vi "Teleop.vi"(10 "Match Info":T1={"Autonomous Elapsed Seconds"=0.0, "TeleOp Elapsed Seconds"=0.0, "Disabled Elapsed Seconds"=0.0, "Visited Autonomous"=FALSE, "Visited TeleOp"=FALSE, "Visited Disabled"=FALSE, "Autonomous Settings"={"Autonomous Style"=enum."Independent", "VI Refnum"=refnum}}, 11 "Call Context":T2) -> ()   [LabVIEW 2020]
doc: "This VI is called for each TeleOp packet received from the DS where the robot is not disabled. It is often used to read from the joysticks and update I/O or to update setpoints for timed control loops. It should complete and return within 20 milliseconds or it may miss DS packets."
uses:
  <vilib>/Rock Robotics/WPI/DriverStation/WPI_DriverStationDerivedRobotMode.ctl
  <vilib>/Rock Robotics/WPI/DriverStation/WPI_DriverStationMatch Info.ctl
  <vilib>/Rock Robotics/WPI/ThirdParty/Phoenix-LabVIEW/Motor Controller/Controls/CTRE_Phoenix_MotorControl_ControlMode.ctl
  <vilib>/Rock Robotics/Network Tables/NT Write Boolean.vi
  <vilib>/Rock Robotics/Network Tables/NT Read Boolean.vi
  <vilib>/Rock Robotics/Network Tables/NT Read Number.vi
  <vilib>/Rock Robotics/WPI/Utilities/WPI_GetSetVariantRefNum.vi
  TitanLib/Lib/Piston Hold.vi
  <vilib>/Rock Robotics/WPI/Solenoid/WPI_SolenoidSetEnum.vi
  TitanLib/Lib/TitanLib.lvlib
panel:
  out "Sample Slider 0":dbl(slide) scale=0.0..5.0
  out "Sample Boolean 1":bool
  out "Sample Boolean 0":bool
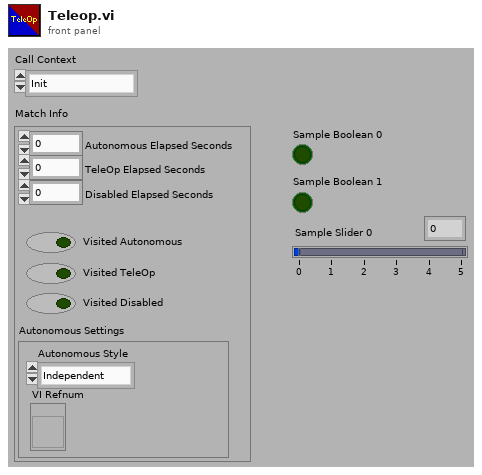
[diagram p1: front panel]
types:
  T1 = typedef "WPI_DriverStationMatch Info.ctl" = cluster{"Autonomous Elapsed Seconds":dbl, "TeleOp Elapsed Seconds":dbl, "Disabled Elapsed Seconds":dbl, "Visited Autonomous":bool, "Visited TeleOp":bool, "Visited Disabled":bool, "Autonomous Settings":cluster{"Autonomous Style":enum16{"Iterative", "Independent"}, "VI Refnum":refnum<vi>}}
  T2 = typedef "WPI_DriverStationDerivedRobotMode.ctl" = enum16{"Init", "Execute", "Stop"}
  T3 = typedef "CTRE_Phoenix_MotorControl_ControlMode.ctl" = u16
  T4 = typedef "WPI_DigitalInputDevRef.ctl" = cluster{"DevStatus":errorcluster, "DIO Channel":T5}
  T5 = typedef "FPGA_DIOChannel.ctl" = enum8{"DIO 0", "DIO 1", "DIO 2", "DIO 3", "DIO 4", "DIO 5", "DIO 6", "DIO 7", "DIO 8", "DIO 9", "DIO MXP 0", "DIO MXP 1", "DIO MXP 2", "DIO MXP 3", "DIO MXP 4", "DIO MXP 5", "DIO MXP 6", "DIO MXP 7", "DIO MXP 8", "DIO MXP 9", "DIO MXP 10", "DIO MXP 11", "DIO MXP 12", "DIO MXP 13", "DIO MXP 14", "DIO MXP 15", "SPI Port CS1", "SPI Port CS2", "SPI Port CS3", "SPI Port MISO", "SPI Port MOSI", "Invalid"}
  T6 = typedef "WPI_JoystickDevRef.ctl" = cluster{"Device":T7}
  T7 = typedef "WPI_JoystickDeviceEnum.ctl" = enum16{"USB 0", "USB 1", "USB 2", "USB 3", "USB 4", "USB 5"}
  T8 = typedef "WPI_MotorControlDeviceRef.ctl" = cluster{"DeviceStatus":errorcluster, "Type":T9, "PWM":cluster{"PWM Channel":T10, "DeadBand":T11}, "CAN":cluster{"Device Number":u8, "SetOutput VI Ref":variant, "GetOutput VI Ref":variant, "Enable VI Ref":variant, "Disable VI Ref":variant, "Data":variant}, "Invert":bool, "DIO PWM":cluster{"PWM \"Enable\" Channel":T10, "DIOChannel":T5, "PWM Rate":dbl}}
  T9 = typedef "WPI_MotorControlType.ctl" = enum16{"PWM", "CAN", "DIO PWM"}
  T10 = typedef "FPGA_DIOPWMChannel.ctl" = enum8{"PWM 0", "PWM 1", "PWM 2", "PWM 3", "PWM 4", "PWM 5", "PWM 6", "PWM 7", "PWM 8", "PWM 9", "PWM MXP 0", "PWM MXP 1", "PWM MXP 2", "PWM MXP 3", "PWM MXP 4", "PWM MXP 5", "PWM MXP 6", "PWM MXP 7", "PWM MXP 8", "PWM MXP 9", "Invalid"}
  T11 = typedef "WPI_PWMDeadband.ctl" = cluster{"Name":string, "maxPositivePwm":i32, "minPositivePwm":i32, "centerPwm":i32, "maxNegativePwm":i32, "minNegativePwm":i32, "angularRange":u16}
  T12 = typedef "WPI_SolenoidValue.ctl" = enum16{"Off", "On", "Forward", "Reverse"}
  T13 = typedef "WPI_SolenoidDevRef.ctl" = cluster{"DevStatus":errorcluster, "Pneumatics Control Module":u8, "Forward Solenoid Channel":T14, "Reverse Solenoid Channel":T14}
  T14 = typedef "WPI_SolenoidChannel.ctl" = enum8{"Solenoid 0", "Solenoid 1", "Solenoid 2", "Solenoid 3", "Solenoid 4", "Solenoid 5", "Solenoid 6", "Solenoid 7", "Solenoid 8", "Solenoid 9", "Solenoid 10", "Solenoid 11", "Solenoid 12", "Solenoid 13", "Solenoid 14", "Solenoid 15", "Invalid"}
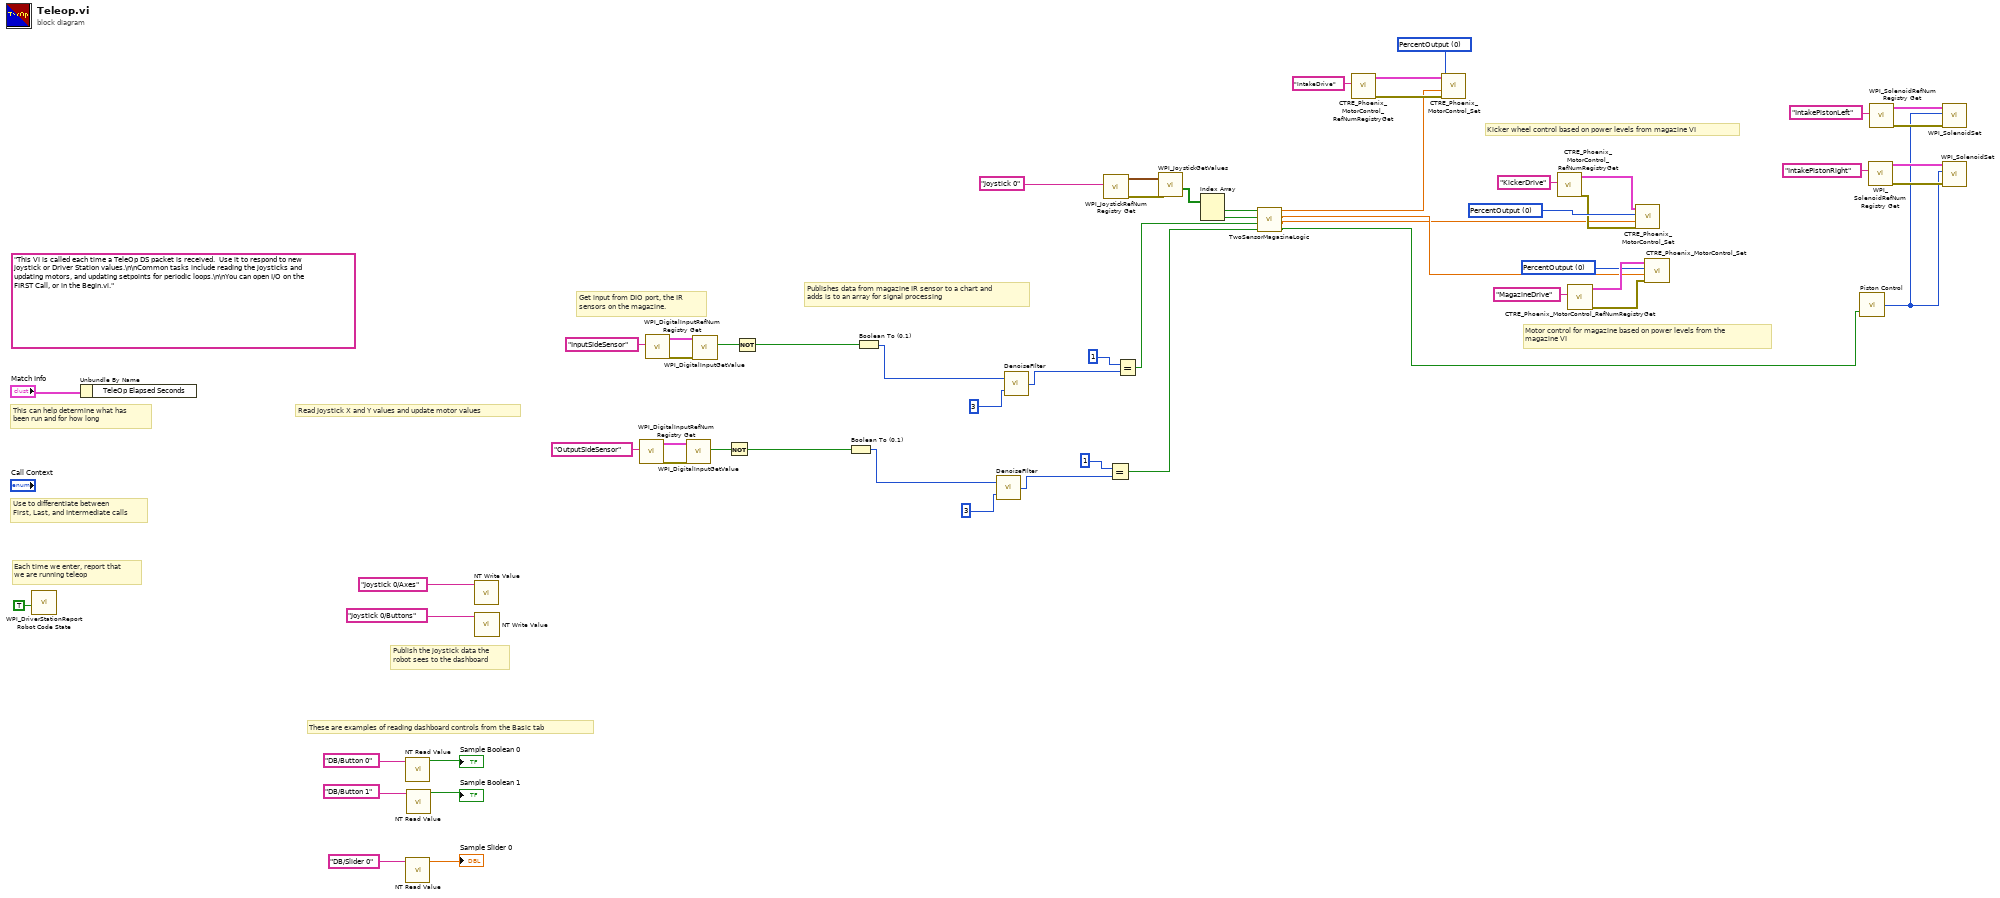
[diagram p0: block diagram]
diagram:
  w26 = T3 0 items=["PercentOutput"=0, "Position"=1, "Velocity"=2, "Current"=3, "Follower"=5, "MotionProfile"=6, "MotionMagic"=7, "MotionProfileArc"=10, "Disabled"=15] ("Control Mode")
  w37 = T3 0 items=["PercentOutput"=0, "Position"=1, "Velocity"=2, "Current"=3, "Follower"=5, "MotionProfile"=6, "MotionMagic"=7, "MotionProfileArc"=10, "Disabled"=15] ("Control Mode")
  w38 = T3 0 items=["PercentOutput"=0, "Position"=1, "Velocity"=2, "Current"=3, "Follower"=5, "MotionProfile"=6, "MotionMagic"=7, "MotionProfileArc"=10, "Disabled"=15] ("Control Mode")
  (unwired) "This VI is called each time a TeleOp DS packet is received.  Use it to respond to new joystick or Driver Station values.\n\nCommon tasks include reading the joysticks and updating motors, and updating setpoints for periodic loops.\n\nYou can open I/O on the FIRST Call, or in the Begin.vi."
  # "Publishes data from magazine IR sensor to a chart and\nadds is to an array for signal processing"
  # "Kicker wheel control based on power levels from magazine VI"
  # "Motor control for magazine based on power levels from the\nmagazine VI"
  # "Get input from DIO port, the IR\nsensors on the magazine."
  # "These are examples of reading dashboard controls from the Basic tab"
  # "Publish the joystick data the\nrobot sees to the dashboard"
  # "Each time we enter, report that\nwe are running teleop"
  # "Use to differentiate between\nFirst, Last, and Intermediate calls"
  # "This can help determine what has\nbeen run and for how long"
  # "Read Joystick X and Y values and update motor values"
  n1 = call <vilib>:"WPI_DriverStationReport Robot Code State.vi"("TeleOp"=TRUE ("Autonomous")) -> ()  [unwired: 10 in, 1 out]
  n2 = Unbundle By Name("Match Info") -> ()  [unwired: 1 out]
  n3 = call-poly <vilib>:"NT Read Value.vi"("Name"="DB/Button 0" ("refnum name")) -> ("Boolean"=→"Sample Boolean 0":bool)  [unwired: 9 in, 1 out]
  n4 = call-poly <vilib>:"NT Read Value.vi"("Name"="DB/Slider 0" ("refnum name")) -> ("Numeric"=→"Sample Slider 0":dbl)  [unwired: 9 in, 1 out]
  n5 = call-poly <vilib>:"NT Read Value.vi"("Name"="DB/Button 1" ("refnum name")) -> ("Boolean"=→"Sample Boolean 1":bool)  [unwired: 9 in, 1 out]
  n6 = call-poly <vilib>:"NT Write Value.vi"("Name"="Joystick 0/Axes") -> ()  [unwired: 10 in, 1 out]
  n7 = call-poly <vilib>:"NT Write Value.vi"("Name"="Joystick 0/Buttons") -> ()  [unwired: 10 in, 1 out]
  n8 = call <vilib>:"WPI_DigitalInputRefNum Registry Get.vi"("refnum name"="OutputSideSensor") -> ("error out"=w44:errorcluster, "DigitalInputDevRef"=w43:T4)  [unwired: 9 in]
  n9 = call <vilib>:"WPI_DigitalInputRefNum Registry Get.vi"("refnum name"="InputSideSensor") -> ("error out"=w46:errorcluster, "DigitalInputDevRef"=w45:T4)  [unwired: 9 in]
  n10 = call <vilib>:"WPI_DigitalInputGetValue.vi"("error in (no error)"=w44, "DigitalInputDevRef"=w43) -> ("Value"=w2:bool)  [unwired: 7 in, 2 out]
  n11 = call <vilib>:"WPI_DigitalInputGetValue.vi"("error in (no error)"=w46, "DigitalInputDevRef"=w45) -> ("Value"=w32:bool)  [unwired: 7 in, 2 out]
  n12 = Not(x=w2) -> (.not. x?=w3:bool)
  n13 = Not(x=w32) -> (.not. x?=w31:bool)
  n14 = Boolean To (0,1)(Boolean=w3) -> (0, 1=w5:i16)
  n15 = Boolean To (0,1)(Boolean=w31) -> (0, 1=w10:i16)
  n16 = call "DenoiseFIlter.vi"("Filter Level"=3, "Singal Input"=w5) -> ("Signal Output"=w7:i16)
  n17 = call "DenoiseFIlter.vi"("Filter Level"=3, "Singal Input"=w10) -> ("Signal Output"=w8:i16)
  n18 = call <vilib>:"WPI_JoystickRefNum Registry Get.vi"("refnum name"="Joystick 0") -> ("error out"=w48:errorcluster, "JoystickDevRef"=w47:T6)  [unwired: 9 in]
  n19 = Equal?(x=i16 1, y=w7) -> (x = y?=w1:bool)
  n20 = Equal?(x=i16 1, y=w8) -> (x = y?=w15:bool)
  n21 = call <vilib>:"WPI_JoystickGetValues.vi"("error in (no error)"=w48, "JoystickDevRef"=w47) -> ("Buttons"=w29:bool[])  [unwired: 5 in, 4 out]
  n22 = Index Array(array=w29) -> (element #1=w17:bool, element #2=w16:bool)  [unwired: 2 in]
  n23 = call "TwoSensorMagazineLogic.vi"("Outtake Side Sensor"=w1, "Intake Side Sensor"=w15, "Outtake Button"=w16, "Intake Toggle"=w17) -> ("Intake Pistons"=w11:bool, "Kicker Motors"=w12:dbl, "Magazine Motors"=w13:dbl, "Intake Motors"=w14:dbl)
  n24 = call <vilib>:"CTRE_Phoenix_MotorControl_RefNumRegistryGet.vi"("refnum name"="IntakeDrive") -> ("error out"=w27:errorcluster, "PhoenixMotorControlDevRef"=w28:T8)  [unwired: 9 in]
  n25 = call <vilib>:"CTRE_Phoenix_MotorControl_Set.vi"("error in (no error)"=w27, "Output"=w14, "Control Mode"=w26, "PhoenixMotorControlDevRef"=w28) -> ()  [unwired: 6 in, 2 out]
  n26 = call <vilib>:"CTRE_Phoenix_MotorControl_RefNumRegistryGet.vi"("refnum name"="KickerDrive") -> ("error out"=w35:errorcluster, "PhoenixMotorControlDevRef"=w36:T8)  [unwired: 9 in]
  n27 = call <vilib>:"CTRE_Phoenix_MotorControl_RefNumRegistryGet.vi"("refnum name"="MagazineDrive") -> ("error out"=w39:errorcluster, "PhoenixMotorControlDevRef"=w40:T8)  [unwired: 9 in]
  n28 = call <vilib>:"CTRE_Phoenix_MotorControl_Set.vi"("error in (no error)"=w35, "Output"=w12, "Control Mode"=w37, "PhoenixMotorControlDevRef"=w36) -> ()  [unwired: 6 in, 2 out]
  n29 = call <vilib>:"CTRE_Phoenix_MotorControl_Set.vi"("error in (no error)"=w39, "Output"=w13, "Control Mode"=w38, "PhoenixMotorControlDevRef"=w40) -> ()  [unwired: 6 in, 2 out]
  n30 = call-poly "Piston Control.vi"("Input"=w11) -> ("Output"=w18:T12)  [unwired: 1 in]
  n31 = call <vilib>:"WPI_SolenoidRefNum Registry Get.vi"("refnum name"="IntakePistonRight") -> ("error out"=w20:errorcluster, "SolenoidDevRef"=w19:T13)  [unwired: 9 in]
  n32 = call <vilib>:"WPI_SolenoidRefNum Registry Get.vi"("refnum name"="IntakePistonLeft") -> ("error out"=w22:errorcluster, "SolenoidDevRef"=w21:T13)  [unwired: 9 in]
  n33 = call-poly <vilib>:"WPI_SolenoidSet.vi"("error in (no error)"=w22, "Value"=w18, "SolenoidDevRef"=w21) -> ()  [unwired: 7 in, 2 out]
  n34 = call-poly <vilib>:"WPI_SolenoidSet.vi"("error in (no error)"=w20, "Value"=w18, "SolenoidDevRef"=w19) -> ()  [unwired: 7 in, 2 out]
